vi "configure.vi"(8 "error in (no error)":errorcluster, 11 "DL090430TriggeredExperimentController in":refnum<class "ExperimentControllerDL090430DAQmxTriggered.lvclass">) -> (0 "error out":errorcluster, 3 "DL090430TriggeredExperimentController out":refnum<class "ExperimentControllerDL090430DAQmxTriggered.lvclass">)   [LabVIEW 2010, in "ExperimentControllerDL090430DAQmxTriggered.lvclass"]
doc: "The dynamic dispatch version of this VI loads and displays the configuration file associated with the plug-in object. The user modify and save the configuration data."
uses:
  ExperimentControllerDL090430DAQmxTriggered.lvclass
  mode_enum.ctl
  ExperimentControllerDL090430DAQmxTriggered.lvclass/ExperimentControllerDL090430DAQmxTriggered.ctl
  common/classes/GenericComponent/GenericComponent/GenericComponent.lvclass
panel:
  in  "mode":T1
  out "Configuration":string
  in  "trigger terminal":tag
  in  "edge":i32(ring)=10280 items=["Rising"=10280, "Falling"=10171]
  in  "cancel":bool
  in  "save":bool
  in  "gate line":tag
  # "Configure DL090430TriggeredExperimentController"
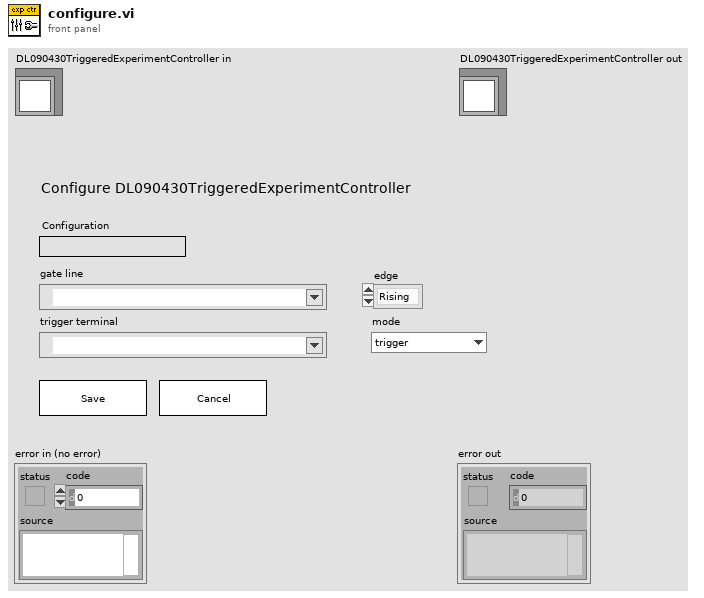
[diagram p1: front panel]
types:
  T1 = typedef "ExperimentControllerDL090430DAQmxTriggered.lvclass/mode_enum.ctl" = enum16{"trigger", "gate"}
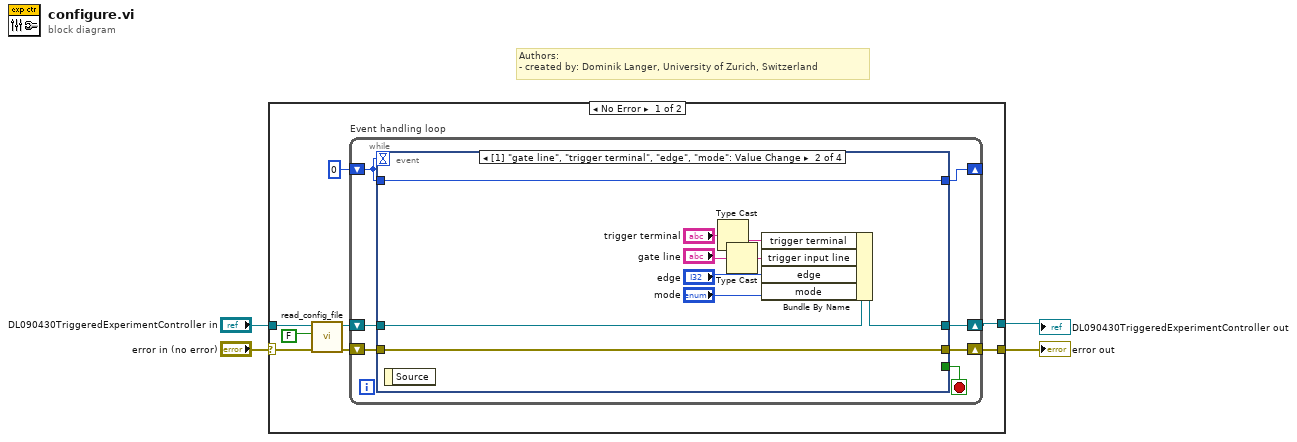
[diagram p0: block diagram]
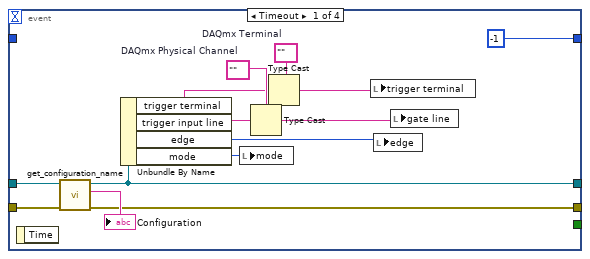
[diagram p2: hidden frame]
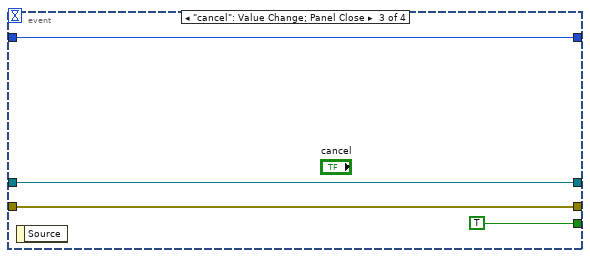
[diagram p3: hidden frame]
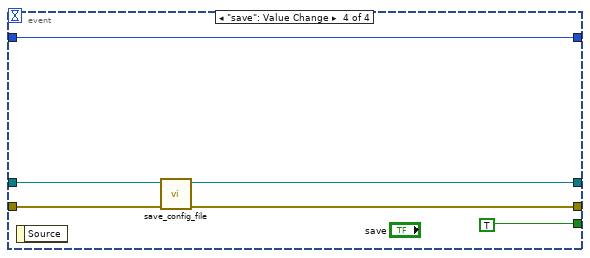
[diagram p4: hidden frame]
diagram:
  # "Authors: \n- created by: Dominik Langer, University of Zurich, Switzerland"
  n1 = case shown="No Error" "error in (no error)" {
    selector: "error in (no error)" -> [w9 w55]
    tunnel: "DL090430TriggeredExperimentController in" -> [w7 w54]
    tunnel: [w12 w55] -> w2
    tunnel: [w11 w54] -> w1
    frame No Error {
      n2 = call-dynamic "read_config_file.vi"("error in (no error)"=w9, "force load?"=FALSE, "GenericPlugin in"=w7) -> ("error out"=w8:errorcluster, "GenericPlugin out"=w6:refnum<class "ExperimentControllerDL090430DAQmxTriggered.lvclass">)  [unwired: 7 out]
      n3 = while "Event handling loop" {
        shift-right: [w16] -> w12
        shift-left: w8 -> [w17]
        shift-right: [w14] -> w11
        shift-left: w6 -> [w15]
        shift-right: [w18] -> _
        shift-left: 0 -> [w19]
        stop <- w13 stop-if-true
        n4 = event shown="[1] \"gate line\", \"trigger terminal\", \"edge\", \"mode\": Value Change" {
          selector: _ -> [_ _ _ _]
          dyn-events: _ -> [_ _ _ _]
          timeout: w19 -> [_ _ _ _]
          tunnel: w19 -> [_ w43 w47 w53]
          tunnel: [-1 w43 w47 w53] -> w18
          tunnel: w17 -> [w24 w42 w46 w51]
          tunnel: [w23 w42 w46 w50] -> w16
          tunnel: w15 -> [w22 w41 w45 w48]
          tunnel: [w21 w40 w45 w49] -> w14
          tunnel: [_ _ TRUE TRUE] -> w13
          event Timeout {
            w26 = tag ""  # DAQmx Terminal
            w29 = tag ""  # DAQmx Physical Channel
            n5 = event-data() -> ()  [unwired: 2 out]
            n6 = call "get_configuration_name.vi"("error in (no error)"=w24, "GenericPlugin.lvclass in"=w22) -> ("error out"=w23:errorcluster, "configuration name"=→"Configuration":string, "GenericPlugin.lvclass out"=w21:refnum<class "ExperimentControllerDL090430DAQmxTriggered.lvclass">)  [unwired: 7 in]
            n7 = Unbundle By Name(w21) -> ("trigger terminal"=w28:string, "trigger input line"=w31:string, "edge"=w32:i32, "mode"=w20:T1)
            n8 = local write "mode"(w20) -> ()
            n9 = Type Cast(type=w29, x=w31) -> (*(type *) &x=w30:tag)
            n10 = Type Cast(type=w26, x=w28) -> (*(type *) &x=w27:tag)
            n11 = local write "trigger terminal"(w27) -> ()
            n12 = local write "edge"(w32) -> ()
            n13 = local write "gate line"(w30) -> ()
          }
          event "gate line", "trigger terminal", "edge": Value Change {
            n14 = event-data() -> ()  [unwired: 2 out]
            n15 = Type Cast(x="trigger terminal") -> (*(type *) &x=w36:string)  [unwired: 1 out]
            n16 = Type Cast(x="gate line") -> (*(type *) &x=w39:string)  [unwired: 1 out]
            n17 = Bundle By Name(cluster=w41, "trigger terminal"=w36, "trigger input line"=w39, "edge"="edge", "mode"="mode") -> (w40:refnum<class "ExperimentControllerDL090430DAQmxTriggered.lvclass">)
          }
          event "cancel": Value Change; Panel Close {
            n18 = event-data() -> ()  [unwired: 2 out]
          }
          event "save": Value Change {
            n19 = event-data() -> ()  [unwired: 2 out]
            n20 = call-dynamic "save_config_file.vi"("error in (no error)"=w51, "GenericPlugin in"=w48) -> ("error out"=w50:errorcluster, "GenericPlugin out"=w49:refnum<class "ExperimentControllerDL090430DAQmxTriggered.lvclass">)  [unwired: 1 in, 7 out]
          }
        }
      }
    }
    frame Error {
    }
  }
  "error out" <- w2
  "DL090430TriggeredExperimentController out" <- w1
